vi "task.vi"   [LabVIEW 2016, in "斯坦道氨氮.lvlib"]
types:
  T1 = enum16{"启动测量", "标样核查", "零点核查", "跨度核查", "空白测试", "平行样测试", "加标回收", "空白校准", "标样校准", "初始化（清洗）", "停止测试", "仪器重启", "校时", "模式设置", "测量间隔设置"}
  T2 = enum16{"启动测量", "标样核查", "零点核查", "跨度核查", "空白测试", "平行样测试", "加标回收", "空白校准", "标样校准", "初始化（清洗）", "停止测试", "仪器重启", "校时", "模式设置", "测量间隔设置"}[]
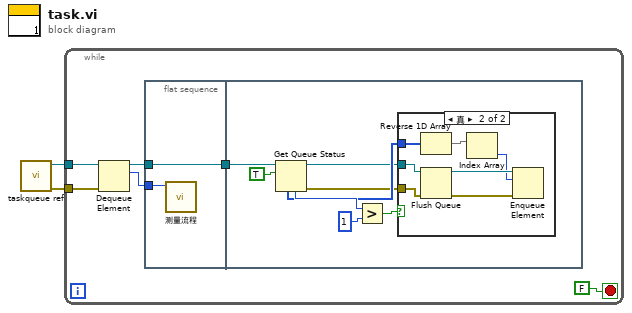
[diagram p0: block diagram]
diagram:
  n1 = call "taskqueue ref.vi"() -> ("错误输出"=w2:errorcluster, "队列输出"=w1:refnum<queue>)  [unwired: 10 in]
  n2 = while {
    tunnel: w1 -> [w7]
    tunnel: w2 -> [w5]
    stop <- FALSE stop-if-true
    n3 = Dequeue Element(queue=w7, error in (no error)=w5) -> (queue out=w4:refnum<queue>, element=w6:T1)  [unwired: 1 in, 2 out]
    n4 = flat-sequence {
      tunnel: w6 -> [w9]
      tunnel: w4 -> [w10]
      tunnel: [w10] -> w3
      tunnel: w3 -> [w18]
      frame #0 {
        n5 = call "测量流程.vi"("控制命令"=w9) -> ()  [unwired: 11 in]
      }
      frame #1 {
        n6 = Get Queue Status(queue=w18, return elements? (F)=TRUE ("返回元素？(F)")) -> (queue out=w13:refnum<queue>, error out=w12:errorcluster, # elements in queue=w16:i32, elements=w14:T2)  [unwired: 1 in, 4 out]
        n7 = Greater?(x=w16, y=1) -> (0:w11:bool)
        n8 = case shown="真" w11 {
          tunnel: w14 -> [_ w25]
          tunnel: w13 -> [_ w23]
          tunnel: w12 -> [_ w22]
          frame False {
          }
          frame True {
            n9 = Reverse 1D Array(array=w25) -> (reversed array=w24:T2)
            n10 = Flush Queue(queue=w23, error in (no error)=w22) -> (queue out=w21:refnum<queue>, error out=w20:errorcluster)  [unwired: 1 out]
            n11 = Index Array(array=w24) -> (element=w19:T1)  [unwired: 1 in]
            n12 = Enqueue Element(queue=w21, element=w19, error in (no error)=w20) -> ()  [unwired: 1 in, 3 out]
          }
        }
      }
    }
  }
